vi "Set Directory Read Only.vi"(4 "error in (no error)":errorcluster, 5 "Recursive":bool, 6 "Make ReadOnly":bool, 7 "Path":path) -> (0 "error out":errorcluster, 3 "Dup Path":path)   [LabVIEW 2011]
panel:
  # "ReadOnly"
  # "Writable"
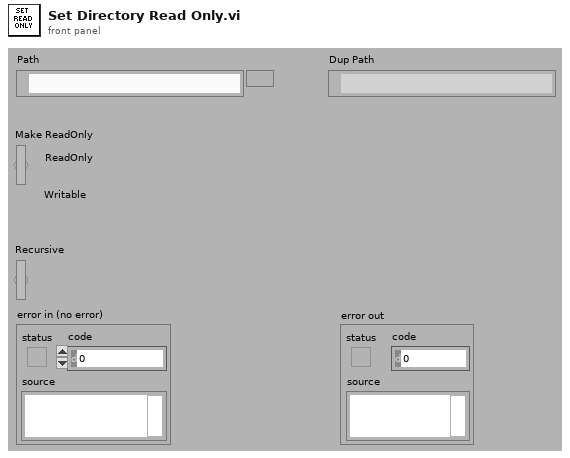
[diagram p1: front panel]
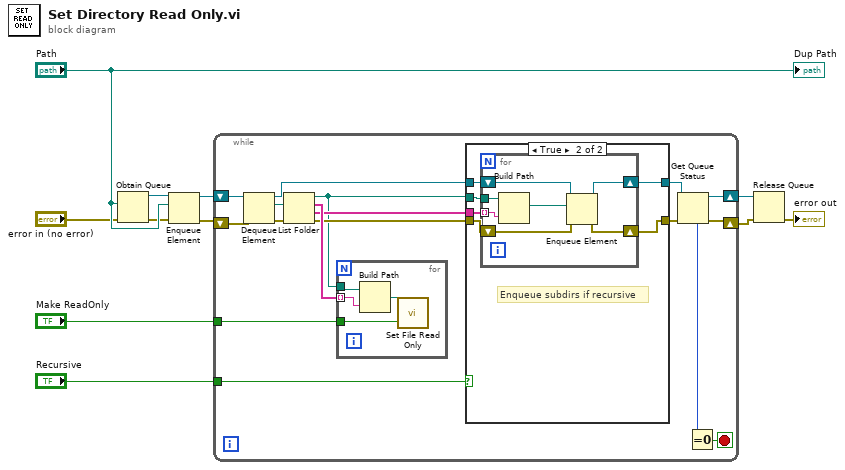
[diagram p0: block diagram]
diagram:
  n1 = Obtain Queue(element data type="Path", error in (no error)="error in (no error)") -> (queue out=w10:refnum<queue>, error out=w7:errorcluster)  [unwired: 2 in, 2 out]
  n2 = Enqueue Element(queue=w10, element="Path", error in (no error)=w7) -> (queue out=w9:refnum<queue>, error out=w6:errorcluster)  [unwired: 2 out]
  n3 = while {
    tunnel: "Make ReadOnly" -> [w28]
    shift-right: [w19] -> w5
    shift-left: w9 -> [w27]
    shift-right: [w20] -> w4
    shift-left: w6 -> [w26]
    tunnel: "Recursive" -> [w18]
    stop <- w22 stop-if-true
    n4 = Dequeue Element(queue=w27, error in (no error)=w26) -> (queue out=w14:refnum<queue>, element=w25:path, error out=w24:errorcluster)  [unwired: 2 out]
    n5 = List Folder(path=w25, error in=w24) -> (path out=w15:path, filenames=w23:string[], folder names=w16:string[], error out=w17:errorcluster)  [unwired: 2 out]
    n6 = for {
      tunnel: w28 -> [w47]
      tunnel: w23 -> [w45] mode=indexing
      tunnel: w15 -> [w46]
      n7 = Build Path(base path=w46, name or relative path=w45) -> (appended path=w44:path)
      n8 = call "Set File Read Only.vi"("Make ReadOnly"=w47, "Path"=w44) -> ()  [unwired: 2 out]
    }
    n9 = case shown="True" w18 {
      tunnel: w17 -> [w29 w33]
      tunnel: w16 -> [_ w36]
      tunnel: w15 -> [_ w35]
      tunnel: w14 -> [w30 w34]
      tunnel: [w29 w32] -> w13
      tunnel: [w30 w31] -> w12
      frame False {
      }
      frame True {
        # "Enqueue subdirs if recursive"
        n10 = for {
          tunnel: w36 -> [w42] mode=indexing
          tunnel: w35 -> [w43]
          shift-right: [w38] -> w31
          shift-left: w34 -> [w41]
          shift-right: [w39] -> w32
          shift-left: w33 -> [w40]
          n11 = Build Path(base path=w43, name or relative path=w42) -> (appended path=w37:path)
          n12 = Enqueue Element(queue=w41, element=w37, error in (no error)=w40) -> (queue out=w38:refnum<queue>, error out=w39:errorcluster)  [unwired: 2 out]
        }
      }
    }
    n13 = Get Queue Status(queue=w12, error in (no error)=w13) -> (queue out=w19:refnum<queue>, error out=w20:errorcluster, # elements in queue=w21:i32)  [unwired: 6 out]
    n14 = Equal To 0?(x=w21) -> (x = 0?=w22:bool)
  }
  n15 = Release Queue(queue=w5, error in (no error)=w4) -> (error out=→"error out":errorcluster)  [unwired: 3 out]
  "Dup Path" <- "Path"
